vi "INI Read write I32.vi"(5 "key":string, 7 "section":string, 8 "error in":errorcluster, 9 "Default":i32, 10 "I32 in":i32, 11 "Read|Write":T1) -> (0 "error out":errorcluster, 2 "I32 out":i32)   [LabVIEW 2013]
doc: "This .vi reads/writes an I32 to the config file. During Write, \"I32 in\" is passed to \"I32 out\""
uses:
  Read write mode.ctl
  <vilib>/Utility/config.llb/Read Key (I32).vi
  <vilib>/Utility/config.llb/Write Key (I32).vi
  <vilib>/Utility/config.llb/NI_LVConfig.lvlib
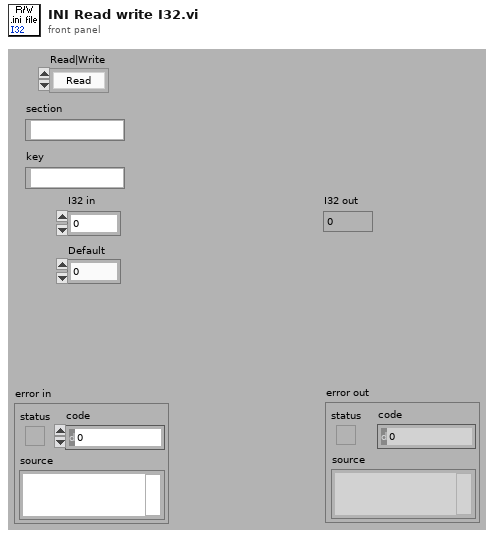
[diagram p1: front panel]
types:
  T1 = typedef "Read write mode.ctl" = enum16{"Read", "Write"}
  T2 = typedef "Semaphore RefNum" = refnum<k1>
  T3 = typedef "NI_LVConfig.lvlib/Config Data RefNum.ctl" = refnum<k1>
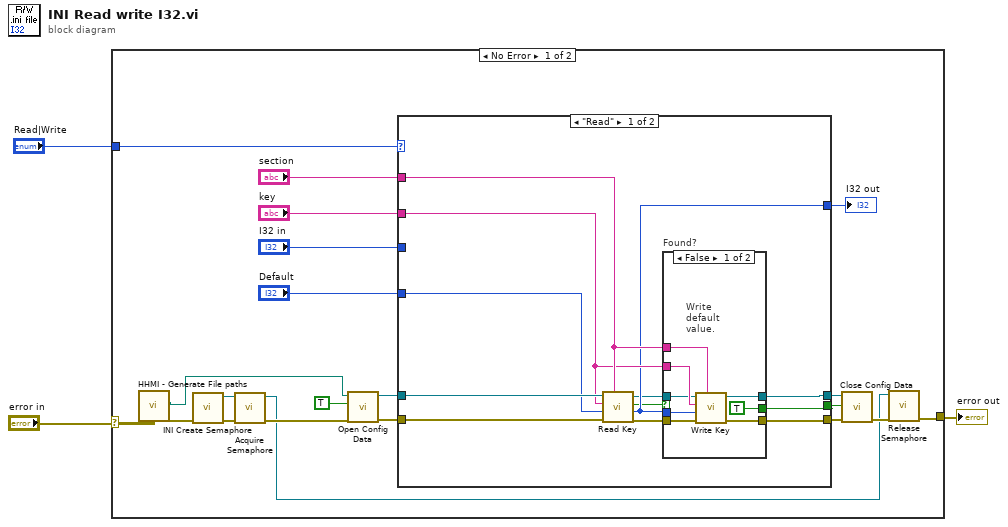
[diagram p0: block diagram]
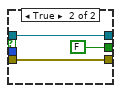
[diagram p2: hidden frame]
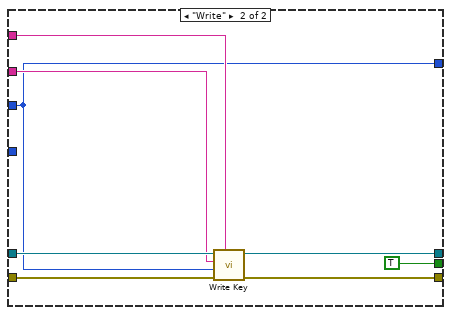
[diagram p3: hidden frame]
diagram:
  n1 = case shown="No Error" "error in" {
    selector: "error in" -> [_ w55]
    tunnel: "Read|Write" -> [w23 _]
    tunnel: [w6 w55] -> w1
    frame No Error {
      n2 = call "HHMI - Generate File paths.vi"() -> ("error out"=w5:errorcluster, ".ini path"=w4:path)  [unwired: 9 in, 1 out]
      n3 = call "INI Create Semaphore.vi"("error in"=w5) -> ("error out"=w11:errorcluster, "semaphore"=w10:T2)  [unwired: 1 in, 4 out]
      n4 = call <vilib>:"Acquire Semaphore.vi"("error in (no error)"=w11, "semaphore"=w10) -> ("error out"=w9:errorcluster, "semaphore out"=w7:T2)  [unwired: 1 in, 3 out]
      n5 = call <vilib>:"Open Config Data.vi"("error in (no error)"=w9, "create file if necessary (T)"=TRUE ("create file if necessary? (T)"), "configuration file path"=w4) -> ("error out"=w18:errorcluster, "refnum"=w21:T3)  [unwired: 6 in, 1 out]
      n6 = case shown="\"Read\"" w23 {
        tunnel: [w31 w53] -> w20
        tunnel: w21 -> [w35 w54]
        tunnel: [w26 w52] -> w19
        tunnel: w18 -> [w34 w51]
        tunnel: "section" -> [w30 w50]
        tunnel: "key" -> [w29 w49]
        tunnel: [w28 w47] -> w15
        tunnel: "I32 in" -> [_ w47]
        tunnel: [w24 TRUE ("write configuration file? (T)")] -> w13
        tunnel: "Default" -> [w33 _]
        frame "Read" {
          n7 = call-poly <vilib>:"Read Key.vi"("section"=w30, "error in (no error)"=w34, "default value"=w33, "key"=w29, "refnum"=w35) -> ("error out"=w32:errorcluster, "value"=w28:i32, "found?"=w27:bool, "refnum out"=w25:T3)  [unwired: 3 out]
          n8 = case "Found?" shown="False" w27 {
            tunnel: w32 -> [w43 w46]
            tunnel: [w42 w46] -> w31
            tunnel: w28 -> [w41 _]
            tunnel: w25 -> [w37 w45]
            tunnel: [w40 w45] -> w26
            tunnel: w30 -> [w39 _]
            tunnel: w29 -> [w38 _]
            tunnel: [TRUE ("write configuration file? (T)") FALSE ("write configuration file? (T)")] -> w24
            frame False {
              # "Write\ndefault\nvalue."
              n9 = call-poly <vilib>:"Write Key.vi"("section"=w39, "error in (no error)"=w43, "value"=w41, "key"=w38, "refnum"=w37) -> ("error out"=w42:errorcluster, "refnum out"=w40:T3)  [unwired: 5 out]
            }
            frame True {
            }
          }
        }
        frame "Write" {
          n10 = call-poly <vilib>:"Write Key.vi"("section"=w50, "error in (no error)"=w51, "value"=w47, "key"=w49, "refnum"=w54) -> ("error out"=w53:errorcluster, "refnum out"=w52:T3)  [unwired: 5 out]
        }
      }
      "I32 out" <- w15
      n11 = call <vilib>:"Close Config Data.vi"("error in (no error)"=w20, "write file if changed (T)"=w13, "refnum"=w19) -> ("error out"=w8:errorcluster)  [unwired: 8 out]
      n12 = call <vilib>:"Release Semaphore.vi"("error in (no error)"=w8, "semaphore"=w7) -> ("error out"=w6:errorcluster)  [unwired: 5 out]
    }
    frame Error {
    }
  }
  "error out" <- w1
